vi "Read.vi"(7 "Read Type":T1, 8 "error in (no error)":errorcluster, 11 "NetworkStreamReader in":refnum<class "NetworkStreamReader.lvclass">) -> (0 "error out":errorcluster, 1 "New element?":bool, 2 "element":variant, 3 "NetworkStreamReader out":refnum<class "NetworkStreamReader.lvclass">, 4 "Time Stamp":timestamp)   [LabVIEW 2011, in "NetworkStreamReader.lvclass"]
doc: "Returns the requested value (either the next element available in the buffer or the most recent element). If there are no elements available in the queue, this VI will return the last valid value it returned."
uses:
  NetworkStreamReader.lvclass
  readType.ctl
  NetworkStreamReader.lvclass/NetworkStreamReader.ctl
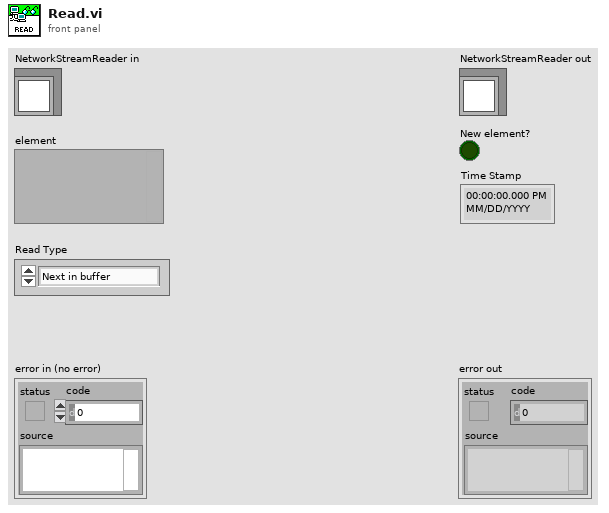
[diagram p1: front panel]
types:
  T1 = typedef "NetworkStreamReader.lvclass/readType.ctl" = enum16{"Next in buffer", "Most current"}
  T2 = typedef "message.ctl" = cluster{"Data":variant, "Time since start (s)":dbl}
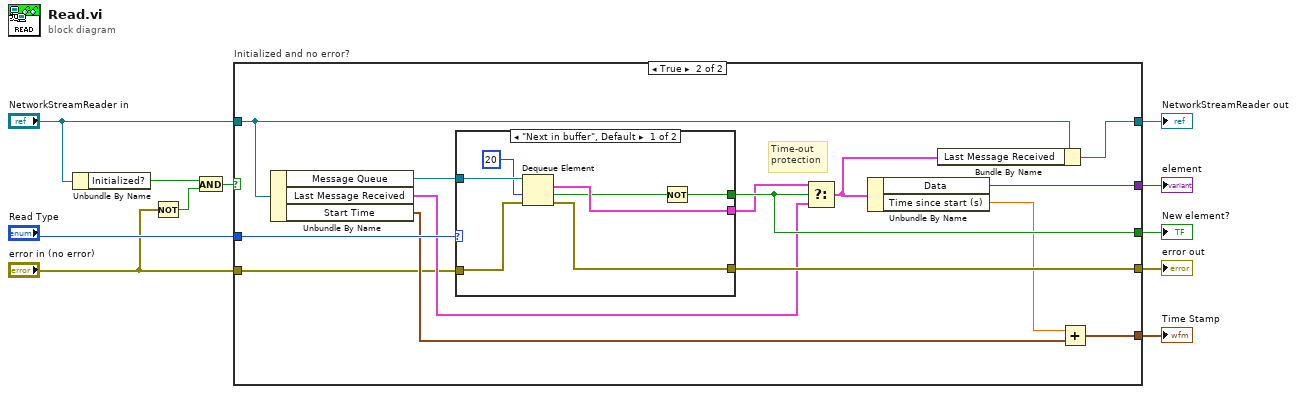
[diagram p0: block diagram]
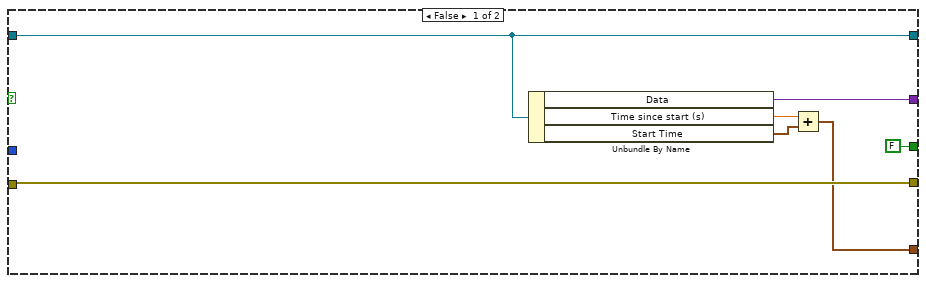
[diagram p2: hidden frame]
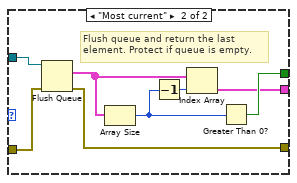
[diagram p3: hidden frame]
diagram:
  n1 = Unbundle By Name("NetworkStreamReader in") -> ("Initialized?"=w1:bool)
  n2 = Not(x="error in (no error)") -> (.not. x?=w2:bool)
  n3 = And(x=w1, y=w2) -> (x .and. y?=w4:bool)
  n4 = case "Initialized and no error?" shown="True" w4 {
    tunnel: [w18 w31] -> w11
    tunnel: [w17 w28] -> w10
    tunnel: "NetworkStreamReader in" -> [w17 w29]
    tunnel: [w16 w23] -> w9
    tunnel: "Read Type" -> [_ w30]
    tunnel: [FALSE w27] -> w7
    tunnel: [w12 w25] -> w6
    tunnel: "error in (no error)" -> [w18 w19]
    frame False {
      n5 = Unbundle By Name(w17) -> ("Data"=w16:variant, "Time since start (s)"=w14:dbl, "Start Time"=w13:timestamp)
      n6 = Add(x=w14, y=w13) -> (x+y=w12:timestamp)
    }
    frame True {
      # "Time-out \nprotection"
      n7 = Unbundle By Name(w29) -> ("Message Queue"=w32:refnum<queue>, "Last Message Received"=w20:T2, "Start Time"=w26:timestamp)
      n8 = case shown="\"Next in buffer\", Default" w30 {
        tunnel: w32 -> [w39 w47]
        tunnel: [w36 w44] -> w31
        tunnel: w19 -> [w37 w46]
        tunnel: [w34 w45] -> w27
        tunnel: [w35 w40] -> w21
        frame "Next in buffer", Default {
          n9 = Dequeue Element(queue=w39, timeout in ms (-1)=20, error in (no error)=w37) -> (element=w35:T2, timed out?=w33:bool, error out=w36:errorcluster)  [unwired: 1 out]
          n10 = Not(x=w33) -> (.not. x?=w34:bool)
        }
        frame "Most current" {
          # "Flush queue and return the last\nelement. Protect if queue is empty."
          n11 = Flush Queue(queue=w47, error in (no error)=w46) -> (remaining elements=w42:T2[], error out=w44:errorcluster)  [unwired: 1 out]
          n12 = Array Size(array=w42) -> (size(s)=w43:i32)
          n13 = Decrement(x=w43) -> (x-1=w41:i32)
          n14 = Index Array(array=w42, index=w41) -> (element=w40:T2)
          n15 = Greater Than 0?(x=w43) -> (x > 0?=w45:bool)
        }
      }
      n16 = Select(t=w21, s=w27, f=w20) -> (s? t:f=w24:T2)
      n17 = Unbundle By Name(w24) -> ("Data"=w23:variant, "Time since start (s)"=w22:dbl)
      n18 = Bundle By Name(cluster=w29, "Last Message Received"=w24) -> (w28:refnum<class "NetworkStreamReader.lvclass">)
      n19 = Add(x=w22, y=w26) -> (x+y=w25:timestamp)
    }
  }
  "error out" <- w11
  "NetworkStreamReader out" <- w10
  "element" <- w9
  "New element?" <- w7
  "Time Stamp" <- w6
